vi "FF_compute.vi"(6 "CenVel":dbl[](array[numeric]), 7 "DesiredM_FF":dbl[](array[numeric])=[5.0, 5.0, 5.0, 4.0, 4.0, 4.0], 10 "CenPt":dbl[](array[numeric]), 11 "Array":T1[](array[typedef])) -> (0 "Closest Pt":dbl[](array[numeric]), 3 "ForceXYZ":dbl[](array[numeric]), 4 "curr Point":dbl[](array[numeric]), 5 "DesiredFM_FF":dbl[](array[numeric]))   [LabVIEW 2013]
uses:
  typeDef/AnkleTraj.ctl
  <vilib>/Analysis/baseanly.llb/Real Dot Product.vi
  <vilib>/Analysis/_algsub.llb/Real Vector Norm.vi
  <vilib>/Analysis/BLAS.llb/idamin - Min Element Index (DBL).vi
  <vilib>/Analysis/NI_AALBase.lvlib
  <vilib>/Analysis/NI_AALPro.lvlib
  <vilib>/Analysis/NI_AALBLAS.lvlib
panel:
  out "P1":dbl[][](array[numeric])
  in  "Array 2":dbl[](array[numeric])=[0.0, 0.05, 0.0]
  in  "Enum":enum16{"Linear", "Bell"}(ring)=enum."Bell"
  out "ForceComp":dbl[](array[numeric])
  out "n_dir":dbl[](array[numeric])
  out "d_min":dbl
  out "TangentVectorAtClosestPt":dbl[](array[numeric])
  out "NormalVectorToClosestPt":dbl[](array[numeric])
  out "DistanceToClosestPt":dbl
  out "IndexOfClosePt":i32
  in  "HalfWindow":i32=60
  in  "Init":bool=TRUE
  # "Mx(Nm)"
  # "My(Nm)"
  # "Mz(Nm)"
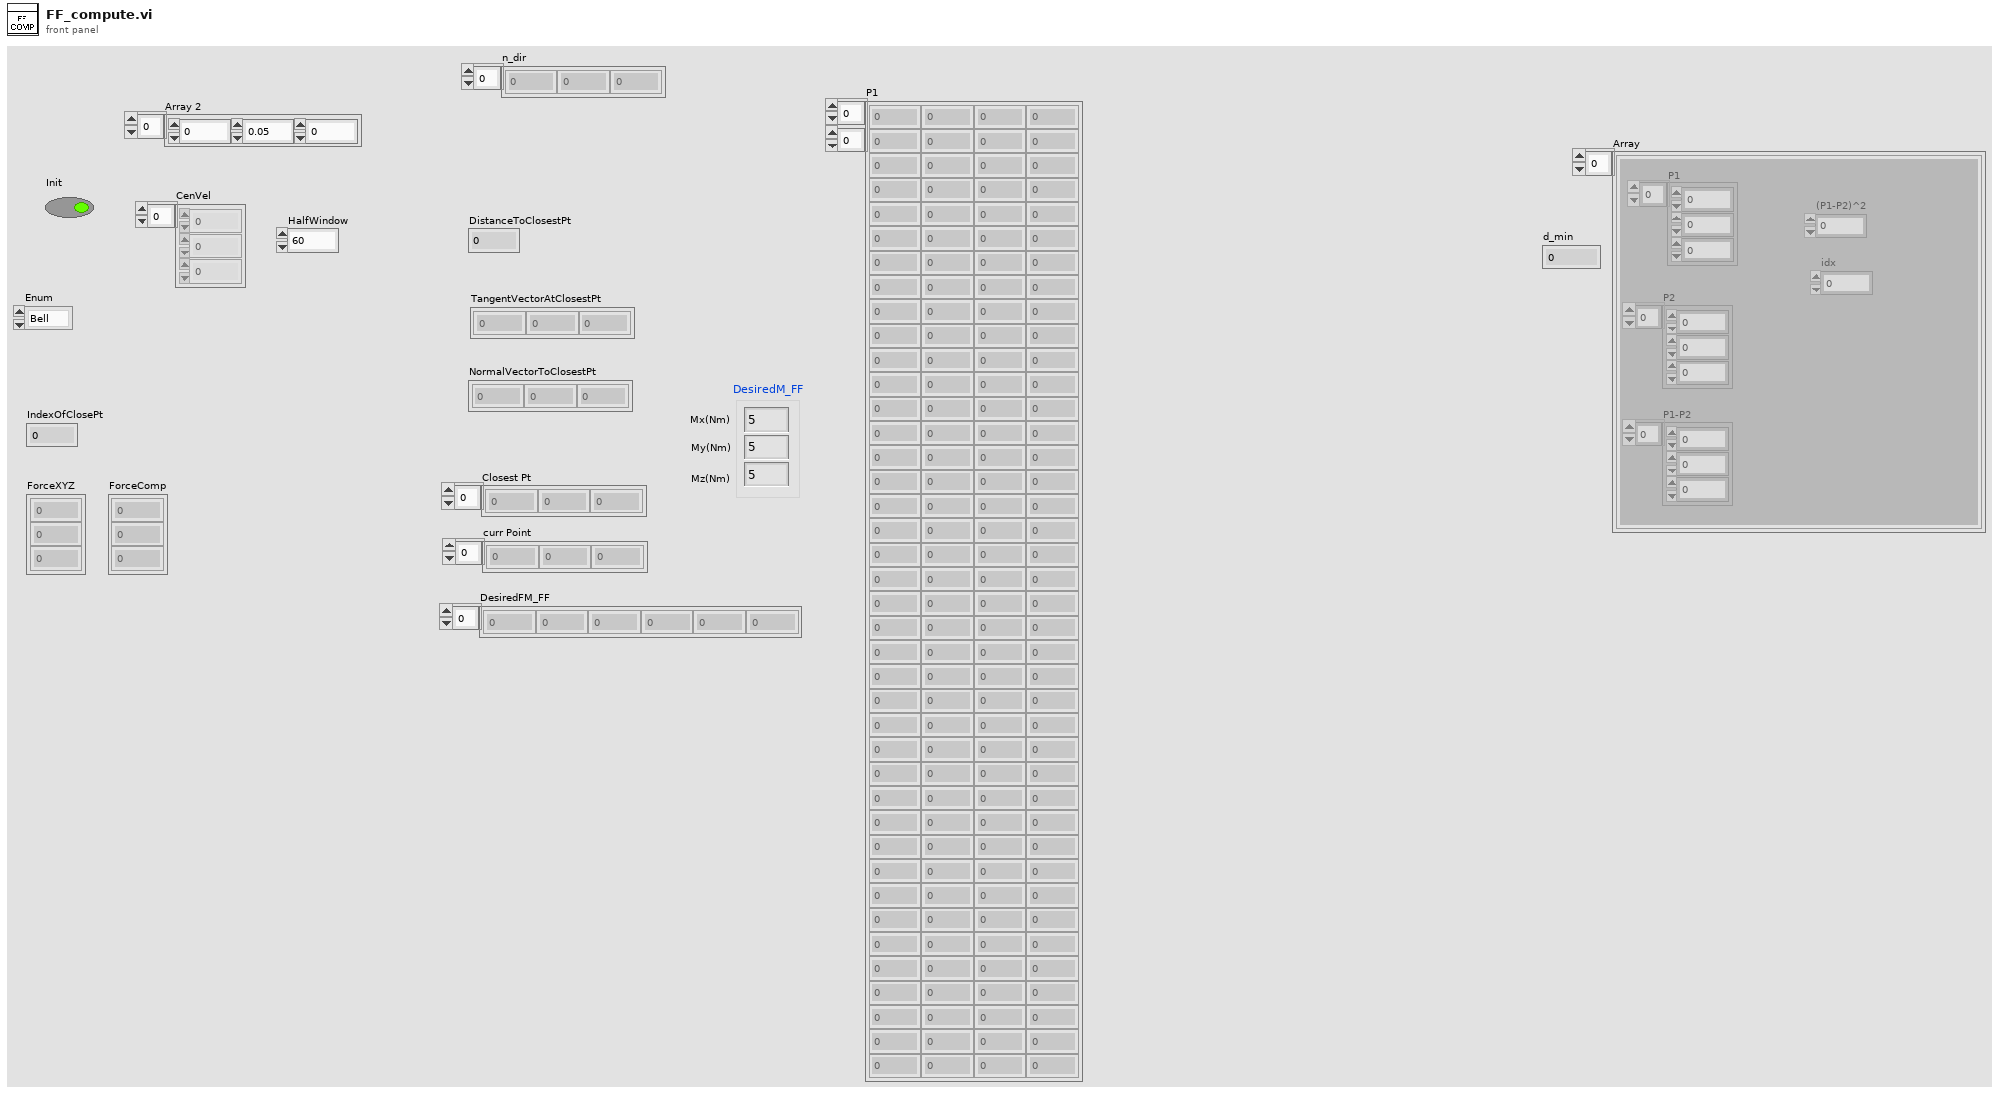
[diagram p1: front panel]
types:
  T1 = typedef "AnkleTraj.ctl" = cluster{"P1":dbl[], "P2":dbl[], "P1-P2":dbl[], "(P1-P2)^2":dbl, "idx":i32}
  T2 = cluster{"Kn":dbl, "Kt":dbl, "Kd":dbl, "Dn":dbl, "Dt":dbl}
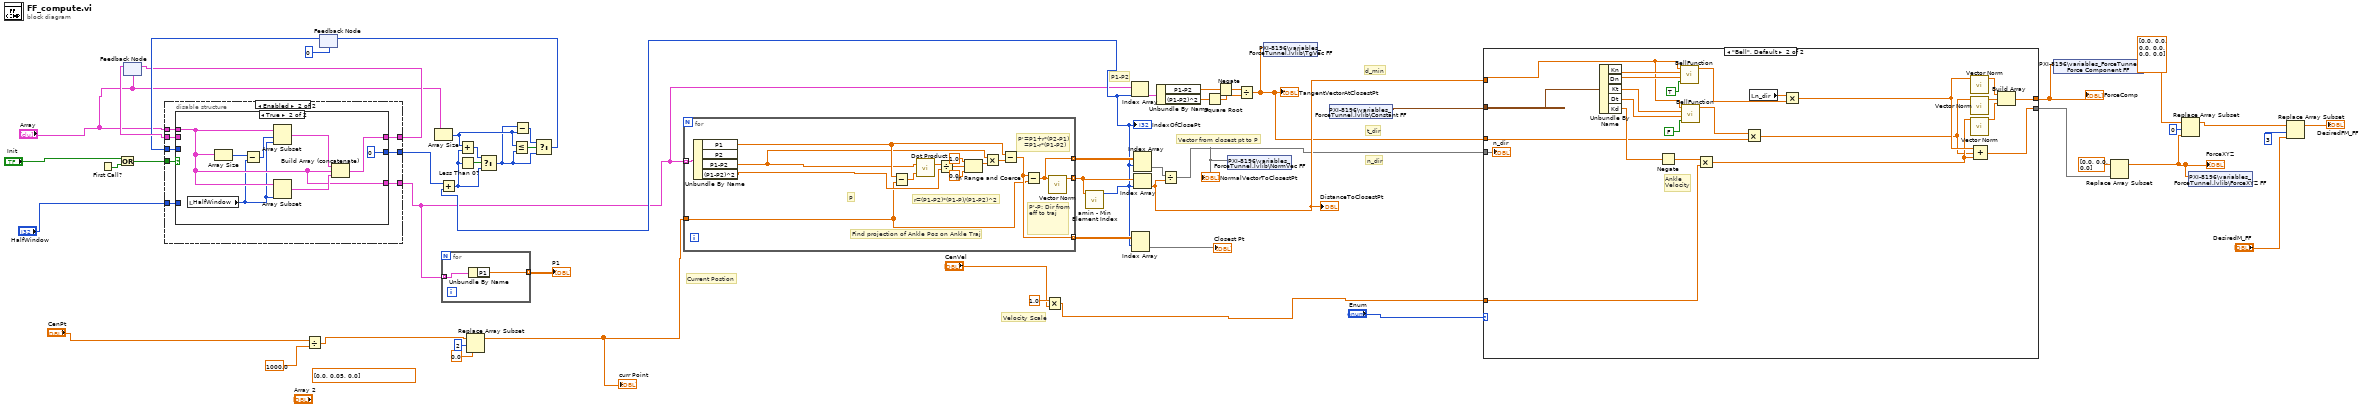
[diagram p0: block diagram]
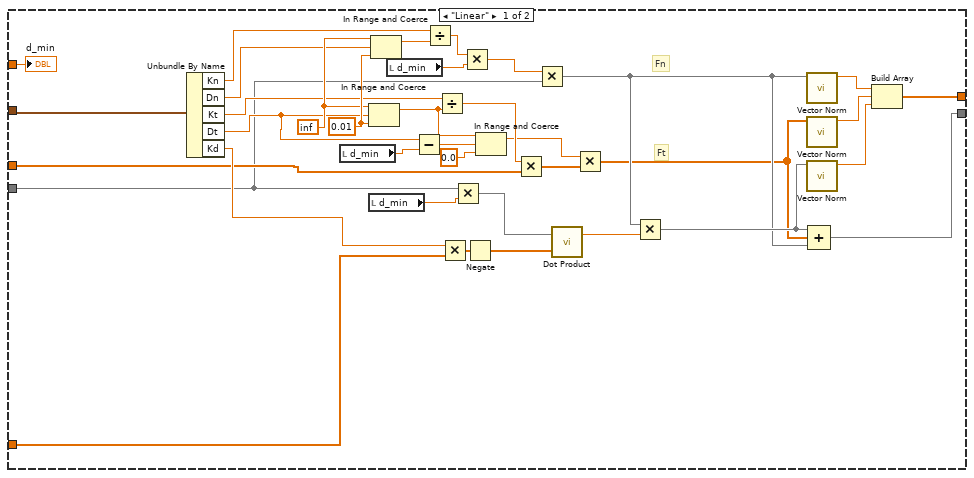
[diagram p2: hidden frame]
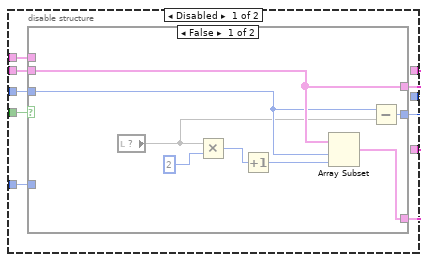
[diagram p3: hidden frame]
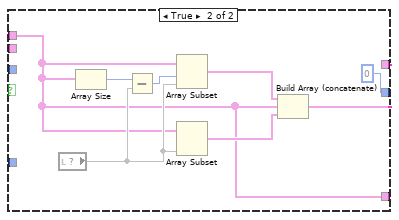
[diagram p4: hidden frame]
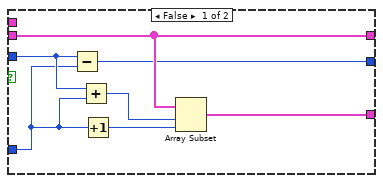
[diagram p5: hidden frame]
diagram:
  (unwired) dbl[] [0.0, 0.05, 0.0]
  # "Current Postion"
  # "Velocity Scale"
  # "P1-P2"
  # "t_dir"
  # "n_dir"
  # "d_min"
  # "Vector from closest pt to P"
  n1 = First Call?() -> (First Call?: T/F=w46:bool)
  n2 = Or(x="Init", y=w46) -> (x .or. y?=w45:bool)
  n3 = feedback #1("Array") -> (w44:T1[])
  n4 = Divide(x="CenPt", y=1000.0) -> (x/y=w13:dbl[])
  n5 = feedback #2(0) -> (w42:i32)
  n6 = disable-structure shown="Enabled" {
    disable-tunnel: w45 -> [w63 w87]
    disable-tunnel: w42 -> [w62 w80]
    disable-tunnel: [w61 w86] -> w8
    disable-tunnel: w44 -> [w60 w81]
    disable-tunnel: [w59 w85] -> w10
    disable-tunnel: [w58 w84] -> w43
    disable-tunnel: "Array" -> [w57 w83]
    disable-tunnel: "HalfWindow" -> [w56 w82]
    frame Disabled {
      n7 = case shown="False" w63 {
        tunnel: w62 -> [w66 _]
        tunnel: w60 -> [w70 _]
        tunnel: [w71 w72] -> w61
        tunnel: [w70 w74] -> w59
        tunnel: [w65 0] -> w58
        tunnel: w57 -> [_ w72]
        tunnel: w56 -> [_ _]
        frame False {
          n8 = local read item#-1() -> (w64)
          n9 = Multiply(x=w64, y=2) -> (x*y=w69:i32)
          n10 = Increment(x=w69) -> (x+1=w68:i32)
          n11 = Array Subset(array=w70, index=w66, length=w68) -> (w71:T1[])
          n12 = Subtract(x=w66, y=w64) -> (x-y=w65:i32)
        }
        frame True {
          n13 = local read item#-1() -> (w78)
          n14 = Array Size(array=w72) -> (size(s)=w79:i32)
          n15 = Subtract(x=w79, y=w78) -> (x-y=w77:i32)
          n16 = Array Subset(array=w72, index=w77, length=w78) -> (w75:T1[])
          n17 = Array Subset(array=w72, length=w78) -> (w76:T1[])  [unwired: 1 in]
          n18 = Build Array (concatenate)(w75, w72, w76) -> (w74:T1[])
        }
      }
    }
    frame Enabled {
      n19 = case shown="True" w87 {
        tunnel: w80 -> [w91 _]
        tunnel: w81 -> [w94 _]
        tunnel: [w88 w96] -> w86
        tunnel: [w94 w98] -> w85
        tunnel: [w92 0] -> w84
        tunnel: w83 -> [_ w96]
        tunnel: w82 -> [w90 _]
        frame False {
          n20 = Subtract(x=w91, y=w90) -> (x-y=w92:i32)
          n21 = Add(x=w91, y=w90) -> (x+y=w89:i32)
          n22 = Increment(x=w90) -> (x+1=w93:i32)
          n23 = Array Subset(array=w94, index=w89, length=w93) -> (w88:T1[])
        }
        frame True {
          n24 = local read "HalfWindow"() -> (w95:i32)
          n25 = Array Size(array=w96) -> (size(s)=w102:i32)
          n26 = Subtract(x=w102, y=w95) -> (x-y=w101:i32)
          n27 = Array Subset(array=w96, index=w101, length=w95) -> (w99:T1[])
          n28 = Array Subset(array=w96, length=w95) -> (w100:T1[])  [unwired: 1 in]
          n29 = Build Array (concatenate)(w99, w96, w100) -> (w98:T1[])
        }
      }
    }
  }
  n30 = feedback-in #1(w10) -> ()
  n31 = Array Size(array="Array") -> (size(s)=w49:i32)
  n32 = for {
    tunnel: w8 -> [w104] mode=indexing
    tunnel: [w103] -> w9 mode=indexing
    n33 = Unbundle By Name(w104) -> ("P1"=w103:dbl[])
  }
  "P1" <- w9
  n34 = Replace Array Subset(array=w13, new element=0.0 ("new element/subarray"), index=2) -> (w22:dbl[])
  "curr Point" <- w22
  n35 = for {
    tunnel: [w112] -> w38 mode=indexing
    tunnel: [w111] -> w39 mode=indexing
    tunnel: [w110] -> w41 mode=indexing
    tunnel: w8 -> [w106] mode=indexing
    tunnel: w22 -> [w105]
    # "P"
    # "P'-P: Dir from eff to traj"
    # "r=(P1-P2)*(P1-P)/(P1-P2)^2"
    # "P'=P1+r*(P2-P1)\n   =P1-r*(P1-P2)"
    # "Find projection of Ankle Pos on Ankle Traj"
    n36 = Unbundle By Name(w106) -> ("P1"=w109:dbl[], "P1-P2"=w108:dbl[], "(P1-P2)^2"=w107:dbl)  [unwired: 1 out]
    n37 = Subtract(x=w109, y=w105) -> (x-y=w119:dbl[])
    n38 = call-poly <vilib>:"Dot Product.vi"("Y Vector"=w119, "X Vector"=w108) -> ("X * Y"=w118:dbl)  [unwired: 1 out]
    n39 = Divide(x=w118, y=w107) -> (x/y=w117:dbl)
    n40 = In Range and Coerce(upper limit=1.0, x=w117, lower limit=0.0) -> (coerced(x)=w114:dbl)  [unwired: 1 out]
    n41 = Multiply(x=w108, y=w114) -> (x*y=w113:dbl[])
    n42 = Subtract(x=w109, y=w113) -> (x-y=w110:dbl[])
    n43 = Subtract(x=w110, y=w105) -> (x-y=w111:dbl[])
    n44 = call-poly <vilib>:"Vector Norm.vi"("Input Vector"=w111) -> ("norm"=w112:dbl)  [unwired: 9 in, 1 out]
  }
  n45 = Multiply(x=1.0, y="CenVel") -> (x*y=w33:dbl[])
  n46 = call-poly <vilib>:"amin - Min Element Index.vi"("x"=w38) -> ("idamin"=w26:i32)  [unwired: 9 in, 1 out]
  "IndexOfClosePt" <- w26
  n47 = Add(x=w43, y=w26) -> (x+y=w47:i32)
  n48 = Add(x=w49, y=w47) -> (x+y=w50:i32)
  n49 = Less Than 0?(x=w47) -> (x < 0?=w51:bool)
  n50 = Select(t=w50, s=w51, f=w47) -> (s? t:f=w48:i32)
  n51 = Less Or Equal?(x=w49, y=w48) -> (x <= y?=w54:bool)
  n52 = Subtract(x=w48, y=w49) -> (x-y=w52:i32)
  n53 = Select(t=w52, s=w54, f=w48) -> (s? t:f=w53:i32)
  n54 = feedback-in #2(w53) -> ()
  n55 = Index Array(array=w8, index=w26) -> (element=w27:T1)
  n56 = Index Array(array=w41, index (row)=w26) -> (element=→"Closest Pt":dbl[])  [unwired: 1 in]
  n57 = Index Array(array=w39, index (row)=w26) -> (element=w40:dbl[])  [unwired: 1 in]
  n58 = Index Array(array=w38, index=w26) -> (element=w34:dbl)
  "DistanceToClosestPt" <- w34
  n59 = Unbundle By Name(w27) -> ("P1-P2"=w30:dbl[], "(P1-P2)^2"=w31:dbl)
  n60 = Divide(x=w40, y=w34) -> (x/y=w2:dbl[])
  "NormalVectorToClosestPt" <- w2
  n61 = Square Root(x=w31) -> (sqrt(x)=w29:dbl)
  n62 = Negate(x=w30) -> (-x=w28:dbl[])
  n63 = shared-variable "PXI-8196\\variables_ForceTunnel.lvlib\\NormVec FF"(w2) -> ()  [unwired: 1 in, 1 out]
  n64 = Divide(x=w28, y=w29) -> (x/y=w1:dbl[])
  "TangentVectorAtClosestPt" <- w1
  n65 = shared-variable "PXI-8196\\variables_ForceTunnel.lvlib\\TgVec FF"(w1) -> ()  [unwired: 1 in, 1 out]
  n66 = shared-variable "PXI-8196\\variables_ForceTunnel.lvlib\\Constant FF"() -> (w4:T2)  [unwired: 1 in, 1 out]
  n67 = case shown="\"Bell\", Default" "Enum" {
    tunnel: [w155 w172] -> w5
    tunnel: [w134 w179] -> w32
    tunnel: w33 -> [w154 w176]
    tunnel: w4 -> [w133 w170]
    tunnel: w1 -> [w127 w161]
    tunnel: w34 -> [w125 w158]
    tunnel: w2 -> [w126 w160]
    frame "Linear" {
      w139 = inf
      w140 = 0.01 ("upper limit")
      # "Ft"
      # "Fn"
      n68 = Unbundle By Name(w133) -> ("Kn"=w132:dbl, "Dn"=w131:dbl, "Kt"=w130:dbl, "Dt"=w129:dbl, "Kd"=w128:dbl)
      n69 = local read "d_min"() -> (w123:dbl)
      n70 = In Range and Coerce(upper limit=w139, x=w129, lower limit=w140) -> (coerced(x)=w141:dbl)  [unwired: 1 out]
      n71 = local read "d_min"() -> (w122:dbl)
      n72 = In Range and Coerce(upper limit=w139, x=w131, lower limit=w140) -> (coerced(x)=w142:dbl)  [unwired: 1 out]
      n73 = local read "d_min"() -> (w124:dbl)
      n74 = Subtract(x=w129, y=w123) -> (x-y=w145:dbl)
      n75 = Divide(x=w132, y=w142) -> (x/y=w138:dbl)
      n76 = Divide(x=w130, y=w141) -> (x/y=w143:dbl)
      n77 = Multiply ("Multiply.vi")(x=w128, y=w154) -> (x*y=w150:dbl[])
      n78 = Multiply(x=w126, y=w122) -> (x*y=w149:dbl[])
      n79 = Multiply(x=w138, y=w124) -> (x*y=w137:dbl)
      n80 = Negate(x=w150) -> (-x=w148:dbl[])
      n81 = In Range and Coerce(upper limit=w141, x=w145, lower limit=0.0) -> (coerced(x)=w120:dbl)  [unwired: 1 out]
      n82 = Multiply(x=w143, y=w127) -> (x*y=w146:dbl[])
      n83 = Multiply(x=w137, y=w126) -> (x*y=w135:dbl[])
      n84 = call-poly <vilib>:"Dot Product.vi"("Y Vector"=w148, "X Vector"=w149) -> ("X * Y"=w147:dbl)  [unwired: 1 out]
      n85 = Multiply(x=w120, y=w146) -> (x*y=w121:dbl[])
      n86 = Multiply(x=w135, y=w147) -> (x*y=w136:dbl[])
      n87 = call-poly <vilib>:"Vector Norm.vi"("Input Vector"=w135) -> ("norm"=w151:dbl)  [unwired: 9 in, 1 out]
      n88 = call-poly <vilib>:"Vector Norm.vi"("Input Vector"=w121) -> ("norm"=w152:dbl)  [unwired: 9 in, 1 out]
      n89 = call-poly <vilib>:"Vector Norm.vi"("Input Vector"=w136) -> ("norm"=w153:dbl)  [unwired: 9 in, 1 out]
      n90 = Compound Arithmetic op=ADD(w136, w121, w135) -> (w134:dbl[])
      n91 = Build Array(w151, w152, w153) -> (w155:dbl[])
      "d_min" <- w125
    }
    frame "Bell", Default {
      # "Ankle\nVelocity"
      n92 = Unbundle By Name(w170) -> ("Kn"=w163:dbl, "Dn"=w164:dbl, "Kt"=w165:dbl, "Dt"=w166:dbl, "Kd"=w169:dbl)
      n93 = Negate(x=w169) -> (-x=w171:dbl)
      n94 = call "BellFunction.vi"("Invert"=TRUE, "(r)adius"=w164, "(A)mplitude"=w163, "x"=w158) -> ("y"=w156:dbl)  [unwired: 2 in]
      n95 = call "BellFunction.vi"("Invert"=FALSE, "(r)adius"=w166, "(A)mplitude"=w165, "x"=w158) -> ("y"=w162:dbl)  [unwired: 2 in]
      n96 = Multiply(x=w171, y=w176) -> (x*y=w177:dbl[])
      n97 = Multiply(x=w162, y=w161) -> (x*y=w157:dbl[])
      n98 = local read "n_dir"() -> (w159:dbl[])
      n99 = Multiply(x=w159, y=w156) -> (x*y=w178:dbl[])
      n100 = call-poly <vilib>:"Vector Norm.vi"("Input Vector"=w178) -> ("norm"=w175:dbl)  [unwired: 9 in, 1 out]
      n101 = call-poly <vilib>:"Vector Norm.vi"("Input Vector"=w157) -> ("norm"=w174:dbl)  [unwired: 9 in, 1 out]
      n102 = call-poly <vilib>:"Vector Norm.vi"("Input Vector"=w177) -> ("norm"=w173:dbl)  [unwired: 9 in, 1 out]
      n103 = Compound Arithmetic op=ADD(w178, w157, w177) -> (w179:dbl[])
      n104 = Build Array(w175, w174, w173) -> (w172:dbl[])
      "n_dir" <- w160
    }
  }
  "ForceComp" <- w5
  n105 = shared-variable "PXI-8196\\variables_ForceTunnel.lvlib\\Force Component FF"(w5) -> ()  [unwired: 1 in, 1 out]
  n106 = Replace Array Subset(array=dbl[] [0.0, 0.0, 0.0], new element=w32) -> (w6:dbl[])  [unwired: 1 in]
  "ForceXYZ" <- w6
  n107 = Replace Array Subset(array=dbl[] [0.0, 0.0, 0.0, 0.0, 0.0, 0.0] ("element"), new element=w6, index=0) -> (w16:dbl[])
  n108 = shared-variable "PXI-8196\\variables_ForceTunnel.lvlib\\ForceXYZ FF"(w6) -> ()  [unwired: 1 in, 1 out]
  n109 = Replace Array Subset(array=w16, new element="DesiredM_FF", index=3) -> (→"DesiredFM_FF":dbl[])
